vi "RichToFlatnixnet_grpc_DbOpenDatabaseRequest.vi"(5 "OutputClusterType":T1, 11 "InputCluster":T3) -> (3 "OutputCluster":T1)   [LabVIEW 2025, in "xnet-grpc_client.lvlib"]
uses:
  xnet-grpc_client.lvlib
  nixnet_grpc_DbOpenDatabaseRequest.ctl
  nidevice_grpc_SessionInitializationBehavior.ctl
  nixnet_grpc_DbOpenDatabaseRequest_Flat.ctl
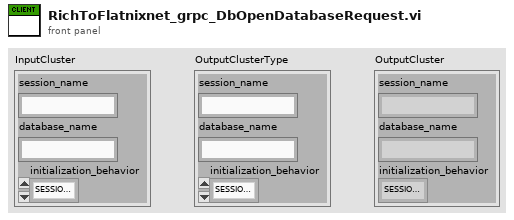
[diagram p1: front panel]
types:
  T1 = typedef "xnet-grpc_client.lvlib/nixnet_grpc_DbOpenDatabaseRequest_Flat.ctl" = cluster{"session_name":string, "database_name":string, "initialization_behavior":T2}
  T2 = typedef "xnet-grpc_client.lvlib/nidevice_grpc_SessionInitializationBehavior.ctl" = enum32{"SESSION_INITIALIZATION_BEHAVIOR_UNSPECIFIED", "SESSION_INITIALIZATION_BEHAVIOR_INITIALIZE_NEW", "SESSION_INITIALIZATION_BEHAVIOR_ATTACH_TO_EXISTING"}
  T3 = typedef "xnet-grpc_client.lvlib/nixnet_grpc_DbOpenDatabaseRequest.ctl" = cluster{"session_name":string, "database_name":string, "initialization_behavior":T2}
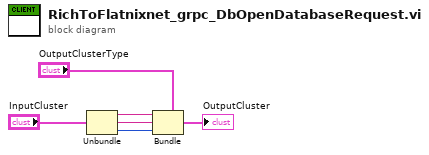
[diagram p0: block diagram]
diagram:
  n1 = Unbundle "Unbundle"("InputCluster") -> ("session_name"=w3:string, "database_name"=w2:string, "initialization_behavior"=w1:T2)
  n2 = Bundle "Bundle"(cluster="OutputClusterType", "session_name"=w3, "database_name"=w2, "initialization_behavior"=w1) -> (→"OutputCluster":T1)
